vi "ph_meter_value _plot.vi"(11 "Numeric":dbl) -> (3 "Waveform Chart":cluster{dbl, "Numeric":dbl, dbl}[](graph))   [LabVIEW 2024]
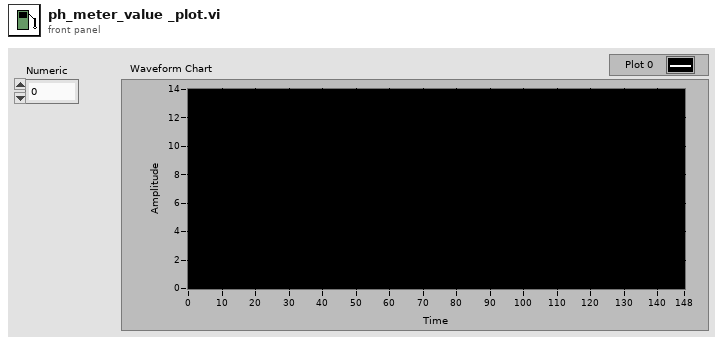
[diagram p1: front panel]
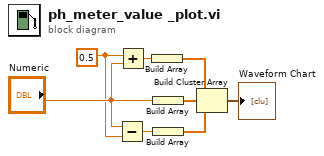
[diagram p0: block diagram]
diagram:
  w7 = 0.5
  n1 = Subtract(x="Numeric", y=w7) -> (x-y=w4:dbl)
  n2 = Add(x=w7, y="Numeric") -> (x+y=w1:dbl)
  n3 = Build Array(w1) -> (w2:dbl[])
  n4 = Build Array("Numeric") -> (w3:dbl[])
  n5 = Build Array(w4) -> (w5:dbl[])
  n6 = Build Cluster Array(w2, w3, w5) -> (→"Waveform Chart":cluster{dbl, "Numeric":dbl, dbl}[])
